vi "Select DB.vi"(8 "error in (no error)":errorcluster, 10 "DB":T1, 11 "Simulated Configuration Database Actor in":refnum<class "Sim Configuration Database Actor.lvclass">) -> (0 "error out":errorcluster, 3 "Simulated Configuration Database Actor out":refnum<class "Sim Configuration Database Actor.lvclass">)   [LabVIEW 2019, in "Sim Configuration Database Actor.lvlib" / "Sim Configuration Database Actor.lvclass"]
uses:
  Sim Configuration Database Actor.lvclass
  DB type.ctl
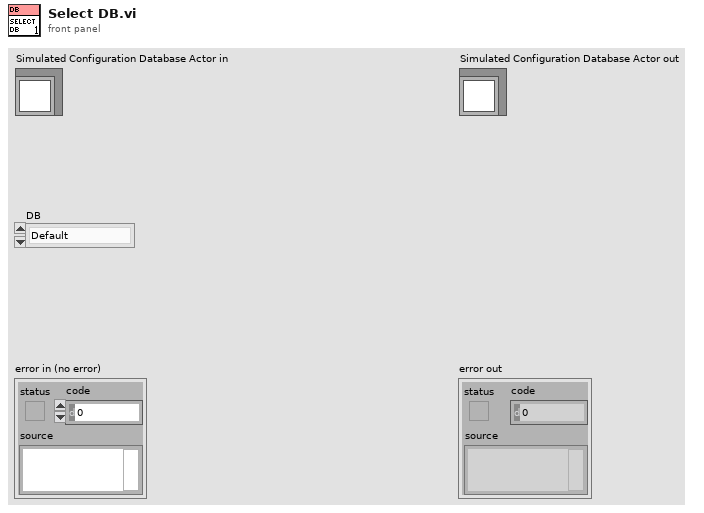
[diagram p1: front panel]
types:
  T1 = typedef "Sim Configuration Database Actor.lvlib/Sim Configuration Database Actor.lvclass/DB type.ctl" = enum16{"Default", "Client"}
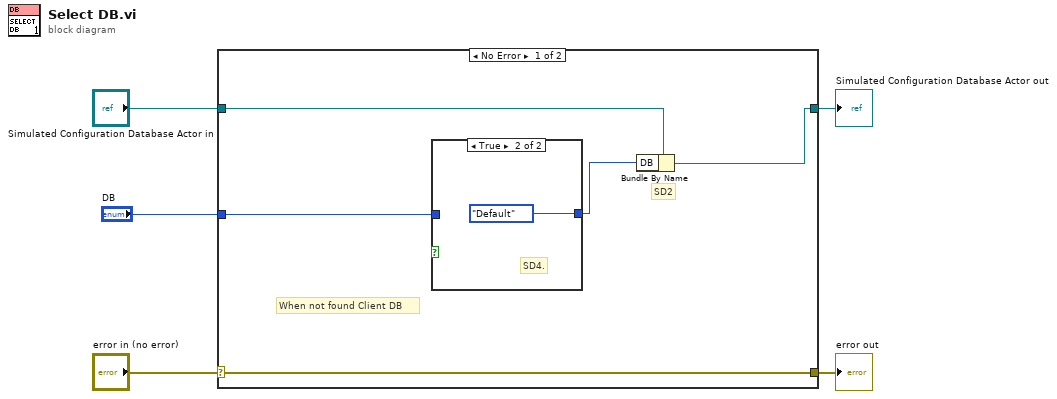
[diagram p0: block diagram]
diagram:
  n1 = case shown="No Error" "error in (no error)" {
    selector: "error in (no error)" -> [w10 w14]
    tunnel: [w10 w14] -> w4
    tunnel: [w7 w13] -> w2
    tunnel: "Simulated Configuration Database Actor in" -> [w9 w13]
    tunnel: "DB" -> [w6 _]
    frame No Error {
      # "When not found Client DB"
      # "SD2"
      n2 = case shown="True" {
        selector: _ -> [_ _]
        tunnel: [w11 DB_type."Default" ("DB")] -> w8
        tunnel: w6 -> [w11 _]
        frame False {
        }
        frame True {
          # "SD4."
        }
      }
      n3 = Bundle By Name(cluster=w9, "DB"=w8) -> (w7:refnum<class "Sim Configuration Database Actor.lvclass">)
    }
    frame Error {
    }
  }
  "error out" <- w4
  "Simulated Configuration Database Actor out" <- w2
